vi "Read EEPROM.vi"(8 "error in (no error)":errorcluster, 9 "Length In":u16, 10 "Offset In":u8, 11 "RTL-SDR in":refnum<class "RTL-SDR.lvclass">) -> (0 "error out":errorcluster, 1 "function return":i32, 2 "Data":u8[](array[numeric]), 3 "RTL-SDR out":refnum<class "RTL-SDR.lvclass">, 4 "Length":u16)   [LabVIEW 2015, in "RTL-SDR.lvclass"]
doc: "Created IvanLis by LabVIEW Portal\nProfile: http://labviewportal.org/memberlist.php?mode=viewprofile&u=987\neMail: IvanLisanov@gMail.com\nTelegram: https://t.me/IvanLis"
uses:
  RTL-SDR.lvclass
  RTL-SDR.lvclass/RTL-SDR.ctl
panel:
  out "Offset":u8
  in  "Data In":u8[](array[numeric])
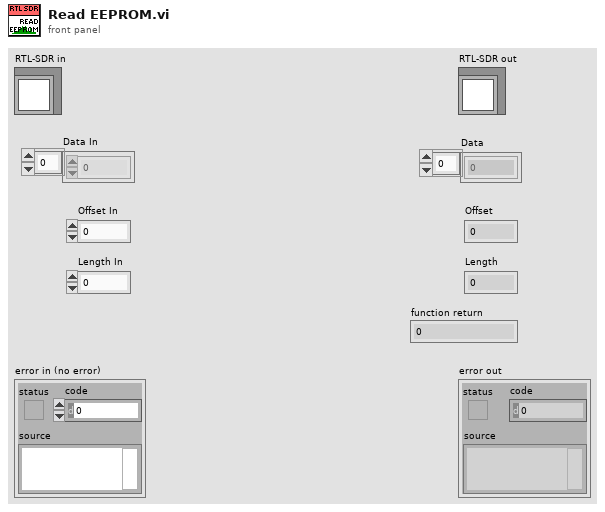
[diagram p1: front panel]
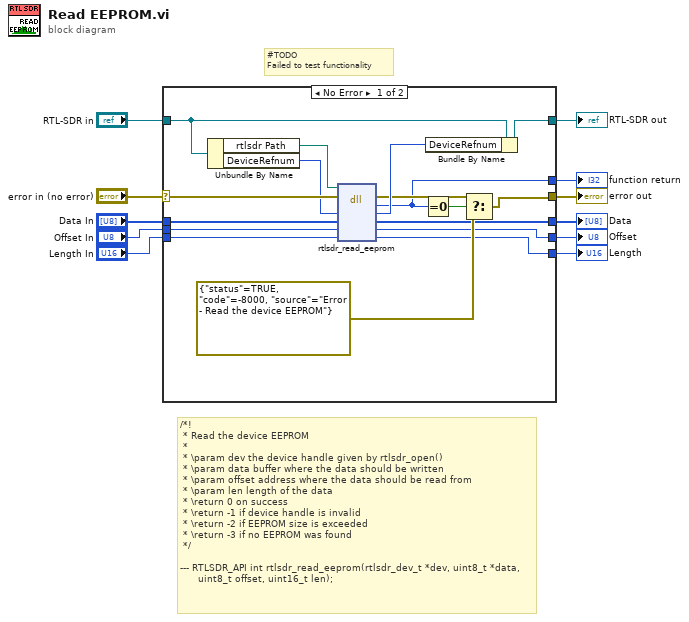
[diagram p0: block diagram]
diagram:
  # "#TODO\nFailed to test functionality"
  # "/*!\n * Read the device EEPROM\n *\n * \\param dev the device handle given by rtlsdr_open()\n * \\param data buffer where the data should be written\n * \\param offset address where the data should be read from\n * \\param len length of the data\n * \\return 0 on success\n * \\return -1 if device handle is invalid\n * \\return -2 if EEPROM size is exceeded\n * \\return -3 if no EEPROM was found\n */\n\n--- RTLSDR_API int rtlsdr_read_eeprom(rtlsdr_dev_t *dev, uint8_t *data,\n\t\t\t\t  uint8_t offset, uint16_t len);"
  n1 = case shown="No Error" "error in (no error)" {
    selector: "error in (no error)" -> [w28 w30]
    tunnel: [w18 w30] -> w10
    tunnel: [w26 w29] -> w8
    tunnel: "RTL-SDR in" -> [w27 w29]
    tunnel: [w17 _] -> w7
    tunnel: "Data In" -> [w16 _]
    tunnel: "Offset In" -> [w22 _]
    tunnel: "Length In" -> [w15 _]
    tunnel: [w14 _] -> w3
    tunnel: [w13 _] -> w2
    tunnel: [w12 _] -> w1
    frame No Error {
      n2 = Unbundle By Name(w27) -> ("rtlsdr Path"=w25:path, "DeviceRefnum"=w24:u64)
      n3 = dll-call lib="C:/Users/Ivan/Desktop/RTL-SDR Class/Project (RTL-SDR)/RTL-SDR Class/dll/rtlsdr.dll" fn="rtlsdr_read_eeprom"(path in=w25, error in=w28, "DeviceRefnum"=w24, "Data"=w16, "Offset"=w22, "Length"=w15) -> (error out=w19:errorcluster, "return type"=w17:i32, "DeviceRefnum"=w23:u64, "Data"=w14:u8[], "Offset"=w13:u8, "Length"=w12:u16)  [unwired: 1 in, 1 out]
      n4 = Equal To 0?(x=w17) -> (x = 0?=w20:bool)
      n5 = Bundle By Name(cluster=w27, "DeviceRefnum"=w23) -> (w26:refnum<class "RTL-SDR.lvclass">)
      n6 = Select(t=w19, s=w20, f=errorcluster {"status"=TRUE, "code"=-8000, "source"="Error - Read the device EEPROM"} ("error out")) -> (s? t:f=w18:errorcluster)
    }
    frame Error {
    }
  }
  "error out" <- w10
  "RTL-SDR out" <- w8
  "function return" <- w7
  "Offset" <- w2
  "Length" <- w1
  "Data" <- w3
